vi "find_image_step_size.vi"(2 "Height":u32, 3 "Width":u32) -> (0 "X Step":u32, 1 "Y Step":u32)   [LabVIEW 2015]
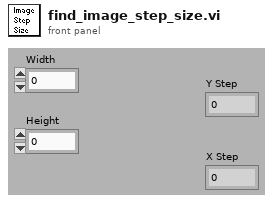
[diagram p1: front panel]
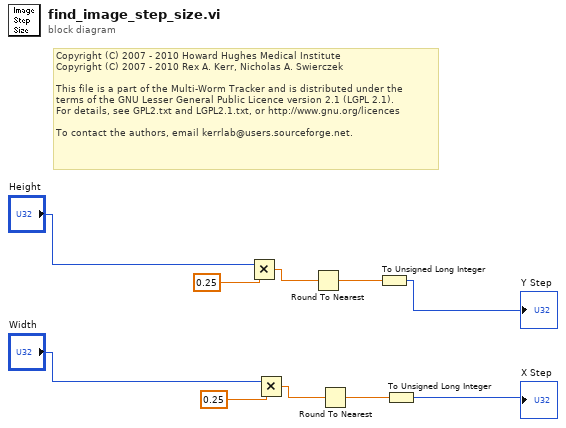
[diagram p0: block diagram]
diagram:
  # "Copyright (C) 2007 - 2010 Howard Hughes Medical Institute\nCopyright (C) 2007 - 2010 Rex A. Kerr, Nicholas A. Swierczek\n \nThis file is a part of the Multi-Worm Tracker and is distributed under the\nterms of the GNU Lesser General Public Licence version 2.1 (LGPL 2.1).\nFor details, see GPL2.txt and LGPL2.1.txt, or http://www.gnu.org/licences\n \nTo contact the authors, email kerrlab@users.sourceforge.net."
  n1 = Multiply(x="Height", y=0.25) -> (x*y=w10:dbl)
  n2 = Multiply(x="Width", y=0.25) -> (x*y=w3:dbl)
  n3 = Round To Nearest(number=w10) -> (nearest integer value=w9:dbl)
  n4 = Round To Nearest(number=w3) -> (nearest integer value=w4:dbl)
  n5 = To Unsigned Long Integer(number=w9) -> (unsigned 32bit integer=→"Y Step":u32)
  n6 = To Unsigned Long Integer(number=w4) -> (unsigned 32bit integer=→"X Step":u32)
